vi "chopperStartStop.vi"(8 "error in (no error)":errorcluster, 10 "start/stop":u16(ring) items=["stop", "start", "ask"], 11 "VISA Refnum in":refnum<visa-resource-name>) -> (0 "error out":errorcluster, 2 "Chopper On?":bool, 3 "VISA Refnum out":refnum<visa-resource-name>)   [LabVIEW 2011]
panel:
  out "read buffer":string
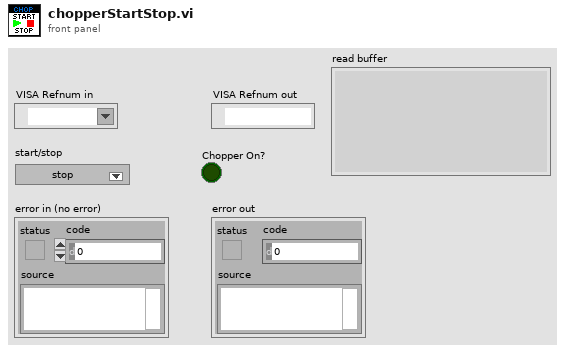
[diagram p1: front panel]
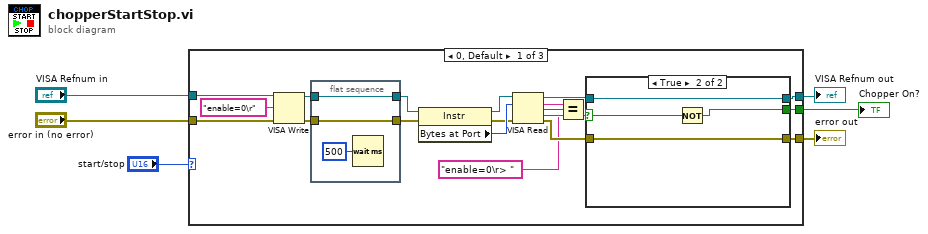
[diagram p0: block diagram]
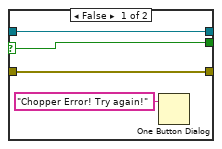
[diagram p2: hidden frame]
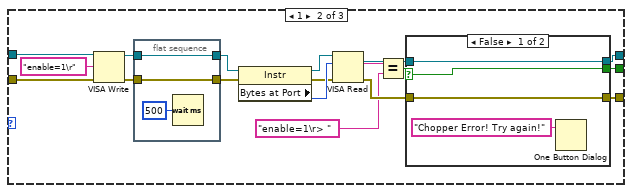
[diagram p3: hidden frame]
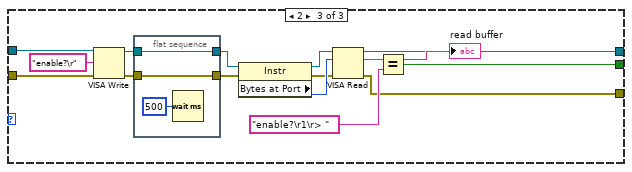
[diagram p5: hidden frame]
diagram:
  n1 = case shown="0, Default" "start/stop" {
    tunnel: "error in (no error)" -> [w24 w53 w78]
    tunnel: "VISA Refnum in" -> [w23 w52 w77]
    tunnel: [w14 w43 w66] -> w6
    tunnel: [w13 w42 w65] -> w5
    tunnel: [w7 w36 w64] -> w1
    frame 0, Default {
      n2 = VISA Write(VISA resource name=w23, write buffer="enable=0\r", error in (no error)=w24) -> (VISA resource name out=w11:refnum<visa-resource-name>, error out=w8:errorcluster)  [unwired: 1 out]
      n3 = flat-sequence {
        tunnel: w11 -> [w27]
        tunnel: [w27] -> w10
        tunnel: [w26] -> w9
        tunnel: w8 -> [w26]
        frame #0 {
          n4 = Wait (ms)(milliseconds to wait=u32 500) -> ()  [unwired: 1 out]
        }
      }
      n5 = property class="Instr"(reference=w10, error in=w9) -> (reference out=w20:refnum<visa-resource-name>, error out=w21:errorcluster, "Bytes at Port"=w22:u32)
      n6 = VISA Read(VISA resource name=w20, byte count=w22, error in (no error)=w21) -> (VISA resource name out=w16:refnum<visa-resource-name>, read buffer=w19:string, error out=w17:errorcluster)  [unwired: 1 out]
      n7 = Equal?(x=w19, y="enable=0\r> ") -> (x = y?=w18:bool)
      n8 = case shown="True" w18 {
        selector: w18 -> [w28 w33]
        tunnel: w17 -> [w30 w34]
        tunnel: w16 -> [w29 w35]
        tunnel: [w29 w35] -> w14
        tunnel: [w30 w34] -> w13
        tunnel: [w28 w32] -> w7
        frame False {
          n9 = One Button Dialog(message="Chopper Error! Try again!") -> ()  [unwired: 1 in, 1 out]
        }
        frame True {
          n10 = Not(x=w33) -> (.not. x?=w32:bool)
        }
      }
    }
    frame 1 {
      n11 = VISA Write(VISA resource name=w52, write buffer="enable=1\r", error in (no error)=w53) -> (VISA resource name out=w40:refnum<visa-resource-name>, error out=w37:errorcluster)  [unwired: 1 out]
      n12 = flat-sequence {
        tunnel: w40 -> [w56]
        tunnel: [w56] -> w39
        tunnel: [w55] -> w38
        tunnel: w37 -> [w55]
        frame #0 {
          n13 = Wait (ms)(milliseconds to wait=u32 500) -> ()  [unwired: 1 out]
        }
      }
      n14 = property class="Instr"(reference=w39, error in=w38) -> (reference out=w49:refnum<visa-resource-name>, error out=w50:errorcluster, "Bytes at Port"=w51:u32)
      n15 = VISA Read(VISA resource name=w49, byte count=w51, error in (no error)=w50) -> (VISA resource name out=w45:refnum<visa-resource-name>, read buffer=w48:string, error out=w46:errorcluster)  [unwired: 1 out]
      n16 = Equal?(x=w48, y="enable=1\r> ") -> (x = y?=w47:bool)
      n17 = case shown="False" w47 {
        selector: w47 -> [w57 w61]
        tunnel: w46 -> [w59 w62]
        tunnel: w45 -> [w58 w63]
        tunnel: [w58 w63] -> w43
        tunnel: [w59 w62] -> w42
        tunnel: [w57 w61] -> w36
        frame False {
          n18 = One Button Dialog(message="Chopper Error! Try again!") -> ()  [unwired: 1 in, 1 out]
        }
        frame True {
        }
      }
    }
    frame 2 {
      n19 = VISA Write(VISA resource name=w77, write buffer="enable?\r", error in (no error)=w78) -> (VISA resource name out=w70:refnum<visa-resource-name>, error out=w67:errorcluster)  [unwired: 1 out]
      n20 = flat-sequence {
        tunnel: w70 -> [w81]
        tunnel: [w81] -> w69
        tunnel: [w80] -> w68
        tunnel: w67 -> [w80]
        frame #0 {
          n21 = Wait (ms)(milliseconds to wait=u32 500) -> ()  [unwired: 1 out]
        }
      }
      n22 = property class="Instr"(reference=w69, error in=w68) -> (reference out=w74:refnum<visa-resource-name>, error out=w75:errorcluster, "Bytes at Port"=w76:u32)
      n23 = VISA Read(VISA resource name=w74, byte count=w76, error in (no error)=w75) -> (VISA resource name out=w66:refnum<visa-resource-name>, read buffer=w73:string, error out=w65:errorcluster)  [unwired: 1 out]
      "read buffer" <- w73
      n24 = Equal?(x=w73, y="enable?\r1\r> ") -> (x = y?=w64:bool)
    }
  }
  "VISA Refnum out" <- w6
  "error out" <- w5
  "Chopper On?" <- w1
